vi "TimeSampleDlg.vi"() -> (1 "定时采样信息":string[][](array[string]), 2 "定时采样信息":T1, 3 "定时采样out":i32(listbox), 5 "是否采样":bool)   [LabVIEW 2014, in "Sample.lvlib"]
uses:
  Sample.lvlib
  DataBase/DataBase.lvlib
  DetectElecrodes/DetectElectros.lvlib
panel:
  out "编号":string
  in  "退出":bool
  in  "删除":bool
  in  "修改":bool
  in  "新增":bool
  in  "定时采样设置":i32(listbox)
  in  "退出":bool
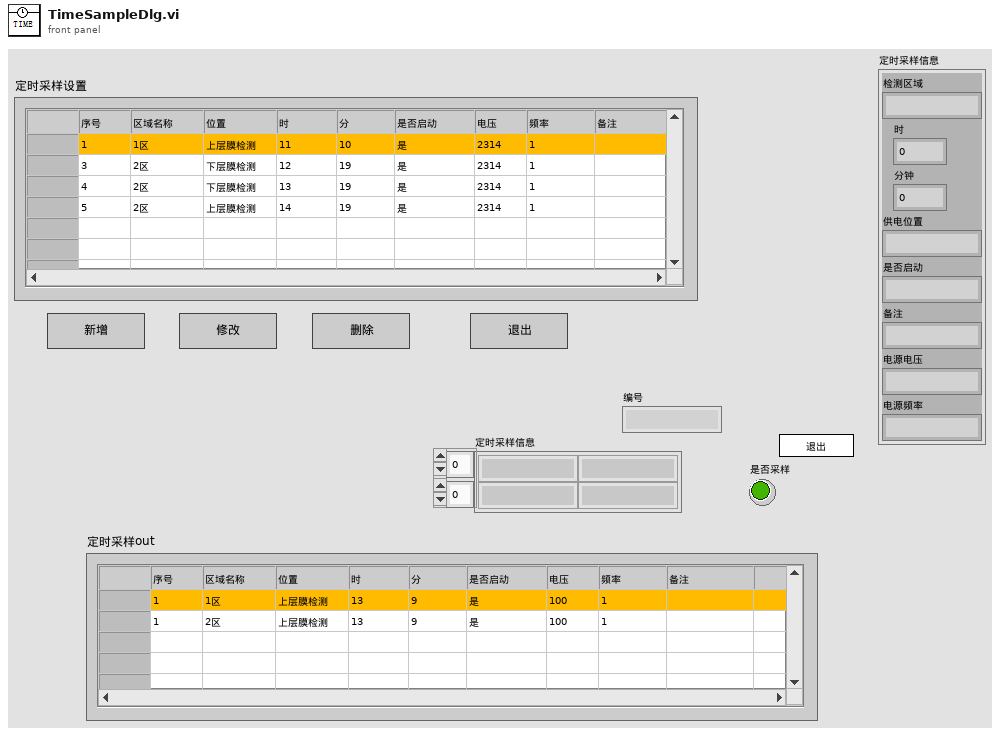
[diagram p1: front panel]
types:
  T1 = cluster{"检测区域":string, "时":u16, "分钟":u16, "供电位置":string, "是否启动":string, "备注":string, "电源电压":string, "电源频率":string}
  T2 = enum32{"invalid app kind", "Development System", "Run Time System", "Student Edition", "Embedded LabVIEW", "Evaluation", "Custom"}
  T3 = enum32{"Invalid", "Standard", "Closed", "Hidden", "Minimized", "Maximized"}
  T4 = cluster{"Core":cluster{"Current VI Reference":refnum<vi>, "Close Panel on Exit?":bool}, "Your Boolean data":bool, "Your string data":string, "定时采样信息":cluster{"检测区域":string, "时":u16, "分钟":u16, "供电位置":string, "是否启动":string, "备注":string, "电源电压":string, "电源频率":string}, "定时采样List":string[], "sampleSet记录":string[][], "Row":i32}
  T5 = typedef "LVPoint32TypeDef.ctl" = cluster{"Horizontal":i32, "Vertical":i32}
  T6 = typedef "LVRowAndColumnTypeDef.ctl" = cluster{"Row":i32, "Column":i32}
  T7 = cluster{"Current VI Reference":refnum<vi>, "Close Panel on Exit?":bool}
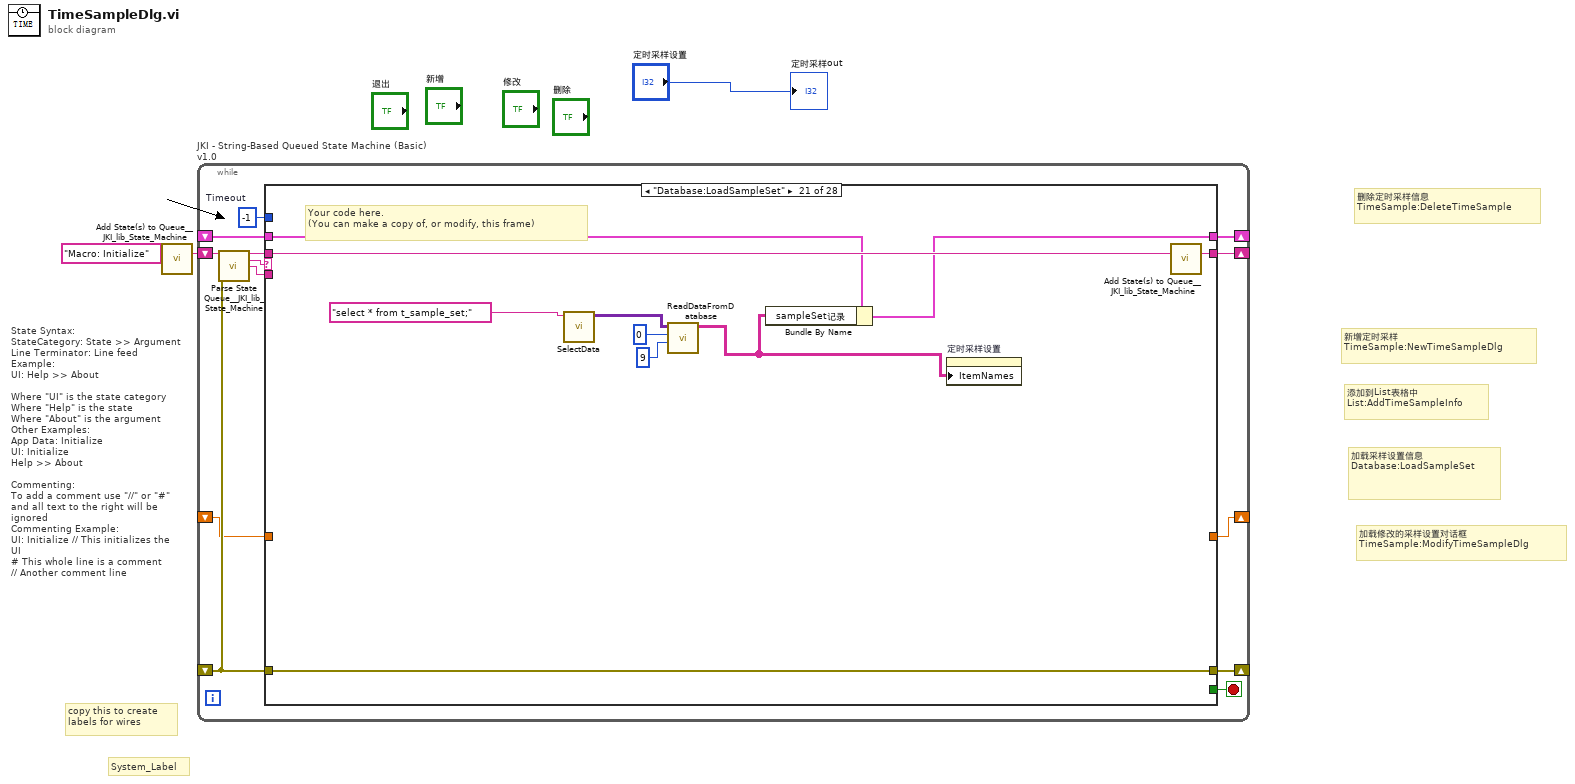
[diagram p0: block diagram]
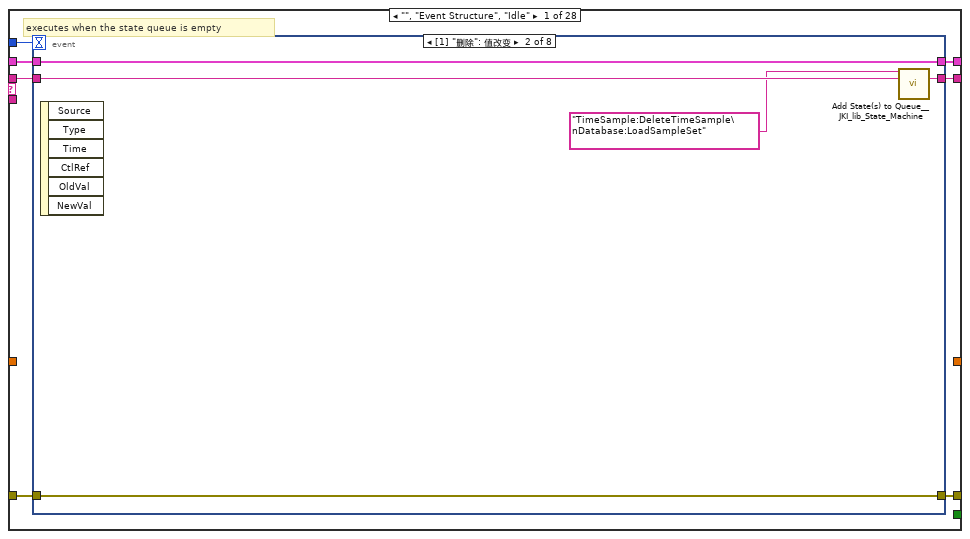
[diagram p2: hidden frame]
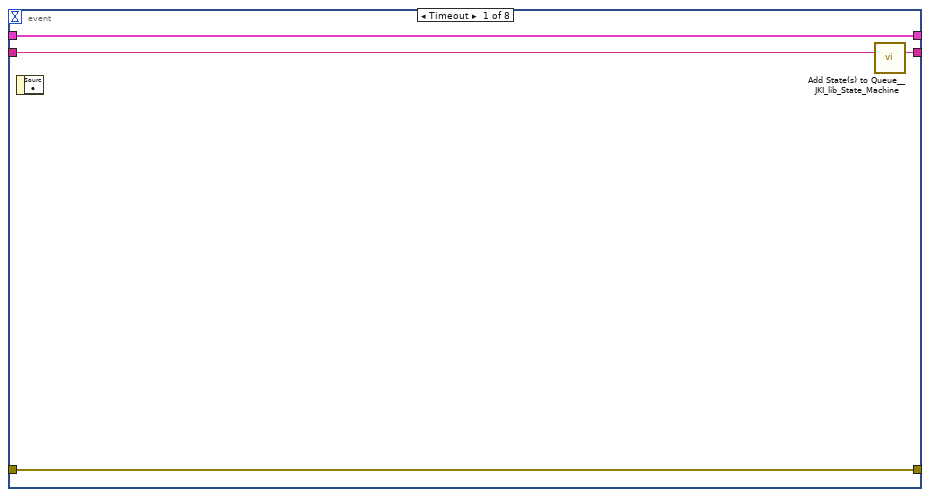
[diagram p3: hidden frame]
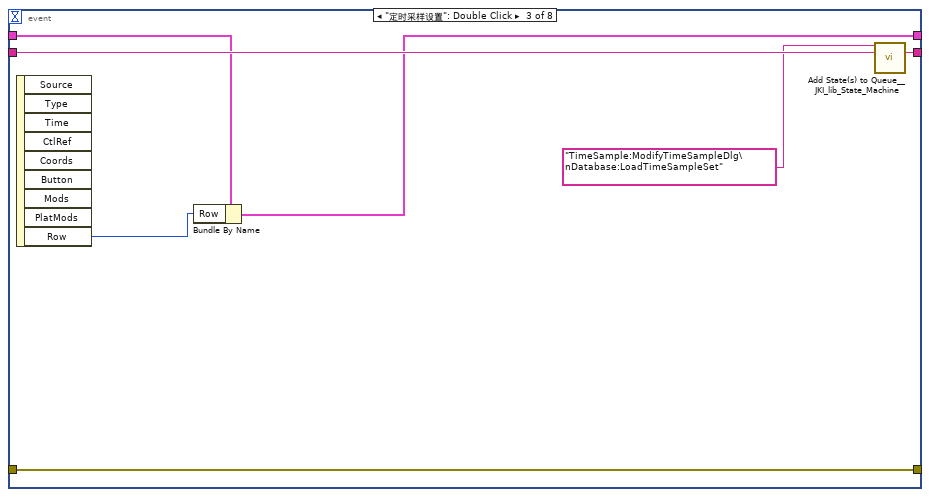
[diagram p4: hidden frame]
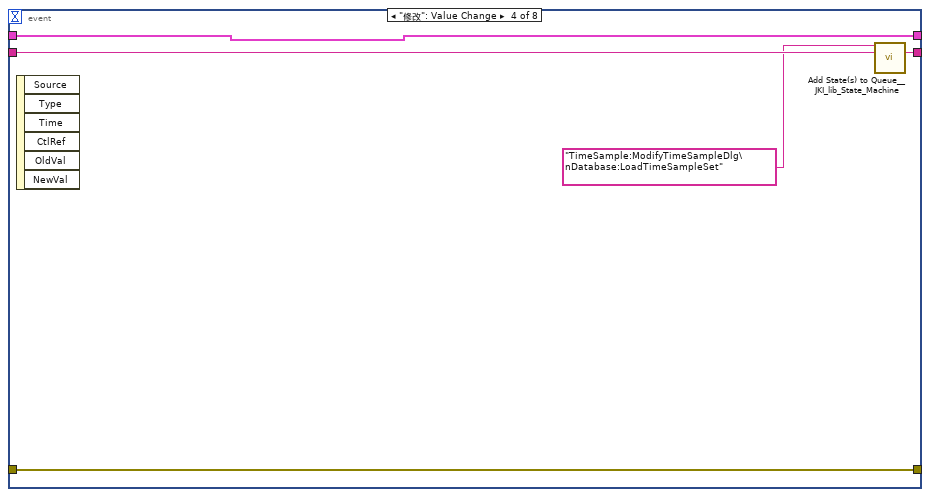
[diagram p5: hidden frame]
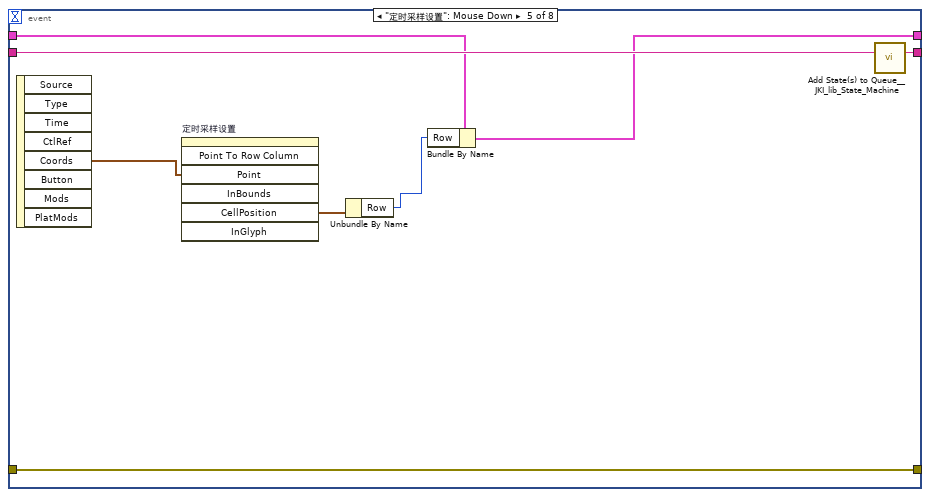
[diagram p6: hidden frame]
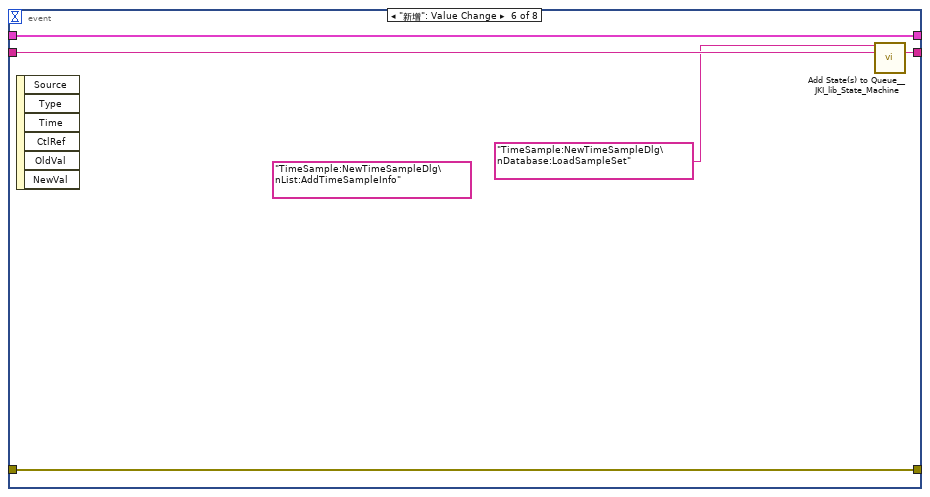
[diagram p7: hidden frame]
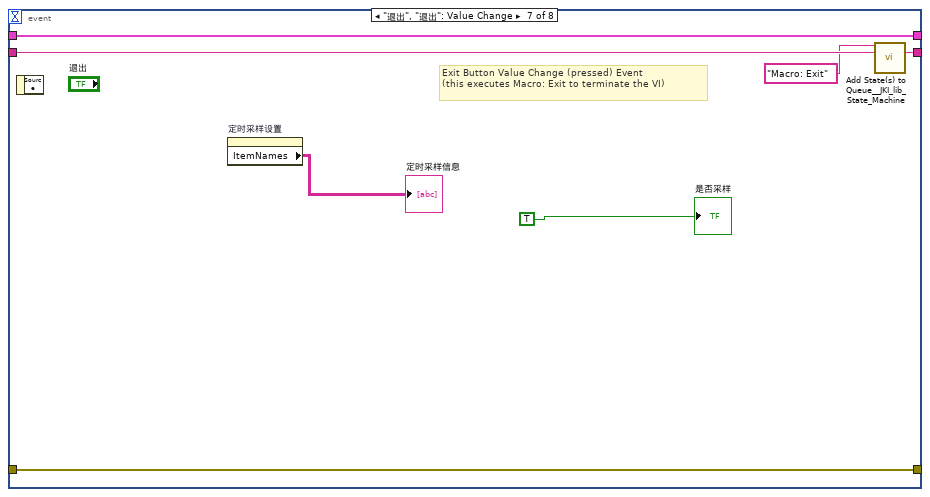
[diagram p8: hidden frame]
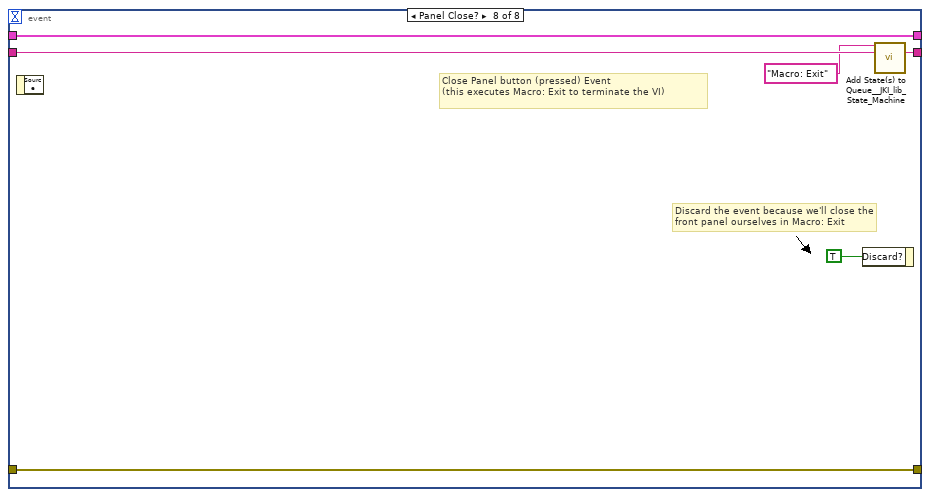
[diagram p9: hidden frame]
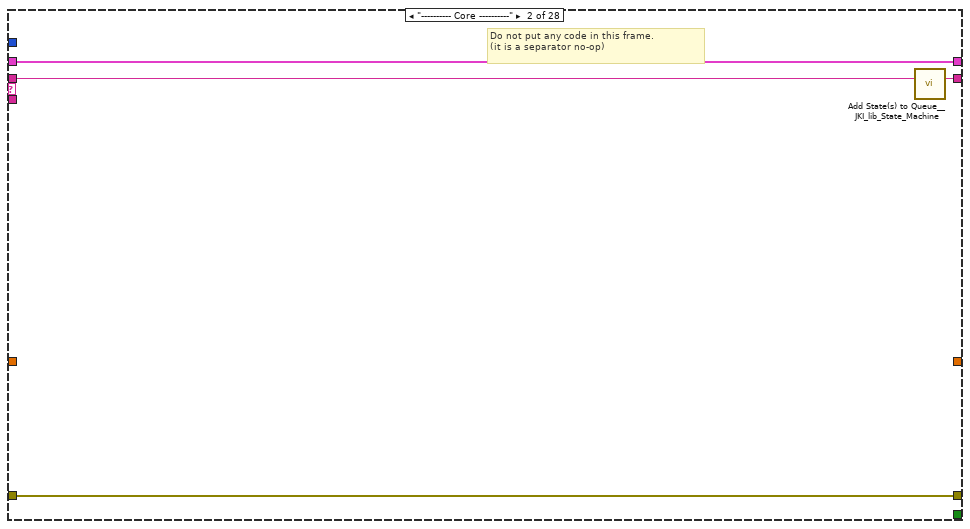
[diagram p10: hidden frame]
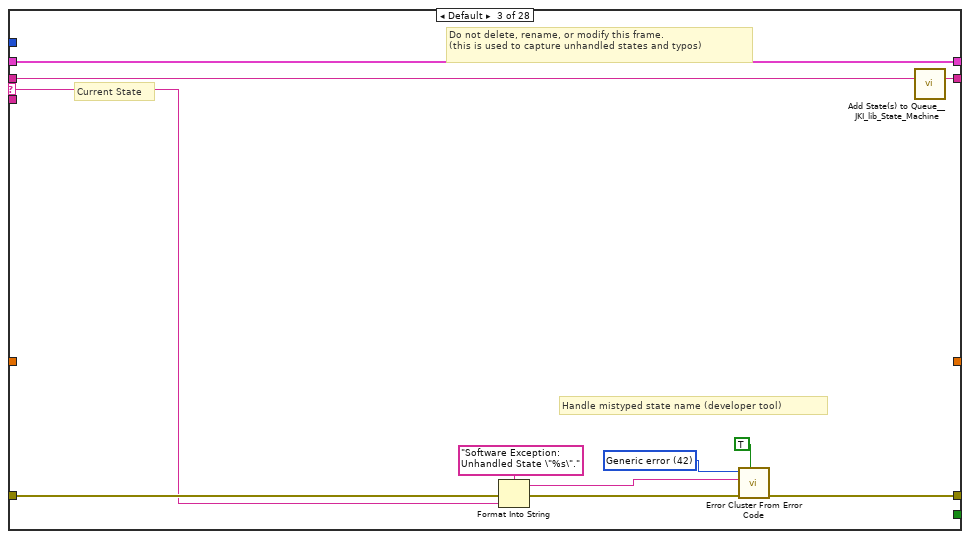
[diagram p11: hidden frame]
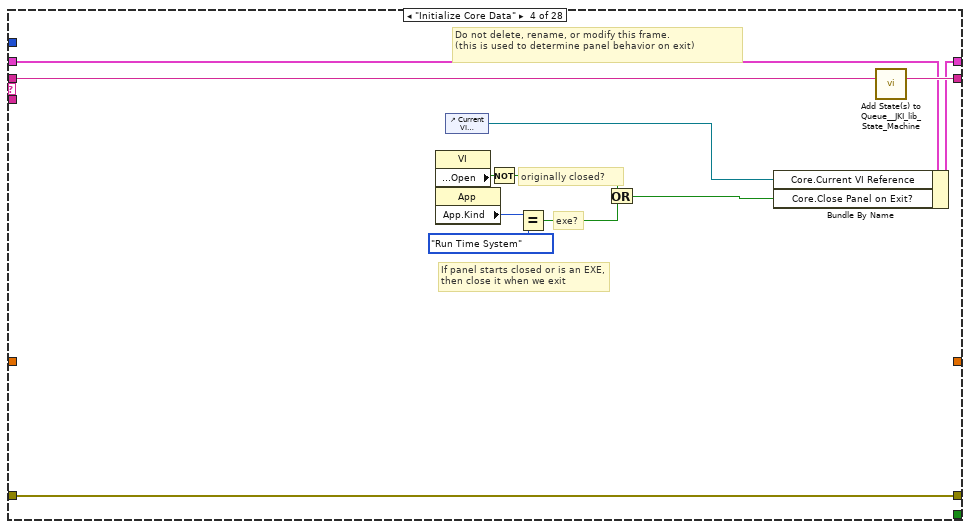
[diagram p12: hidden frame]
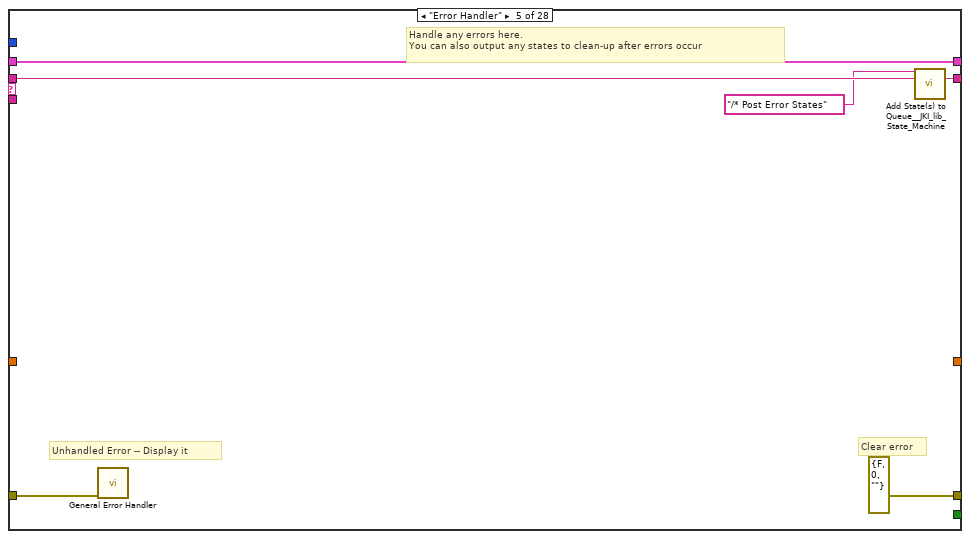
[diagram p13: hidden frame]
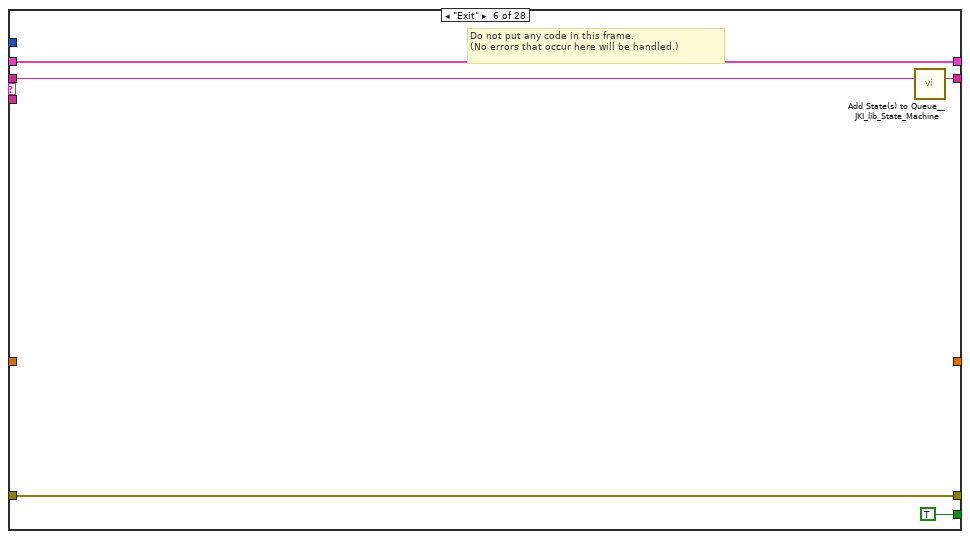
[diagram p14: hidden frame]
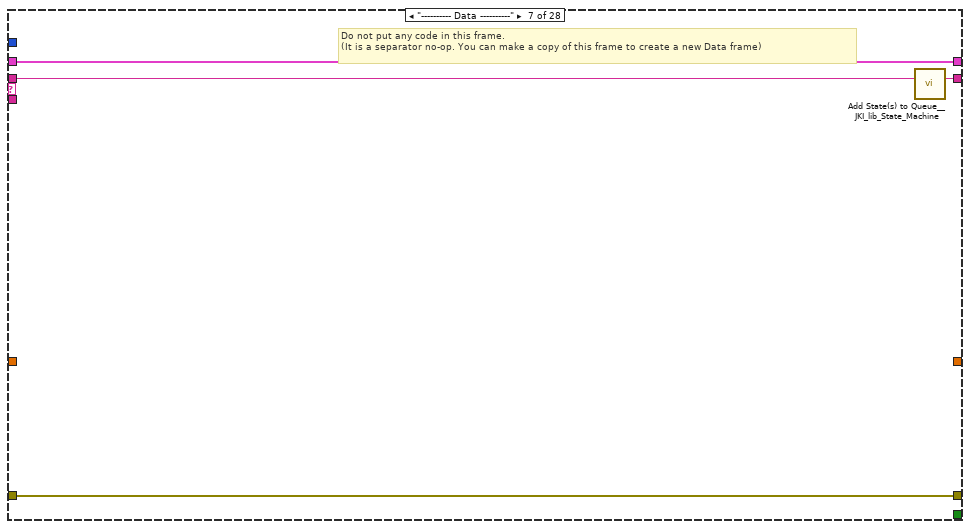
[diagram p15: hidden frame]
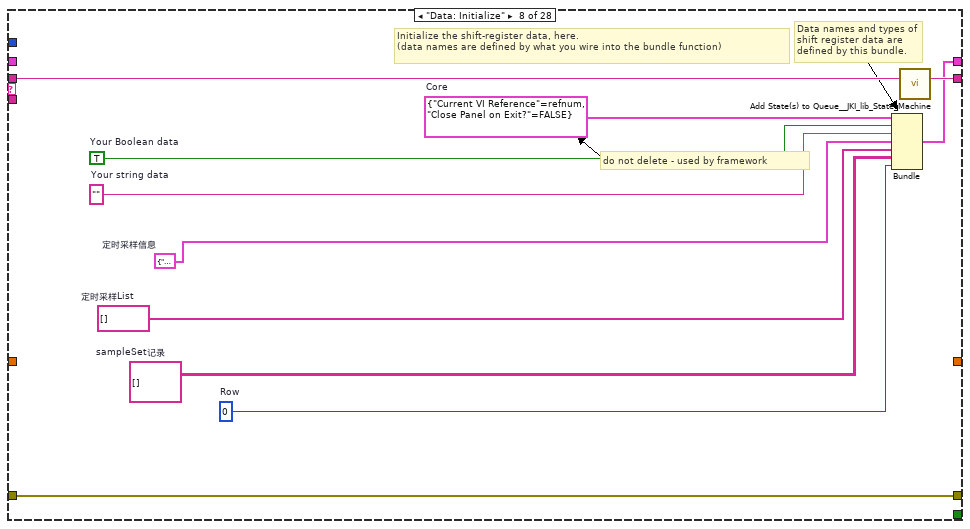
[diagram p16: hidden frame]
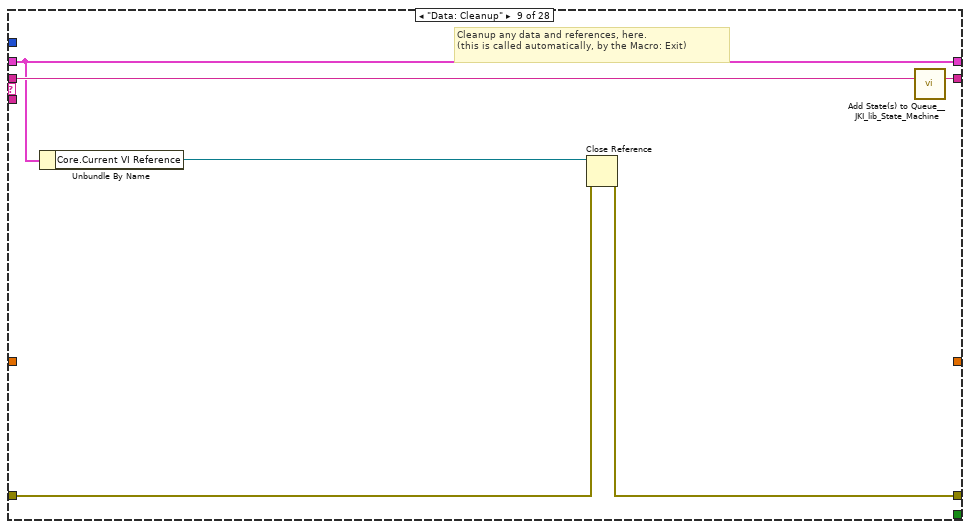
[diagram p17: hidden frame]
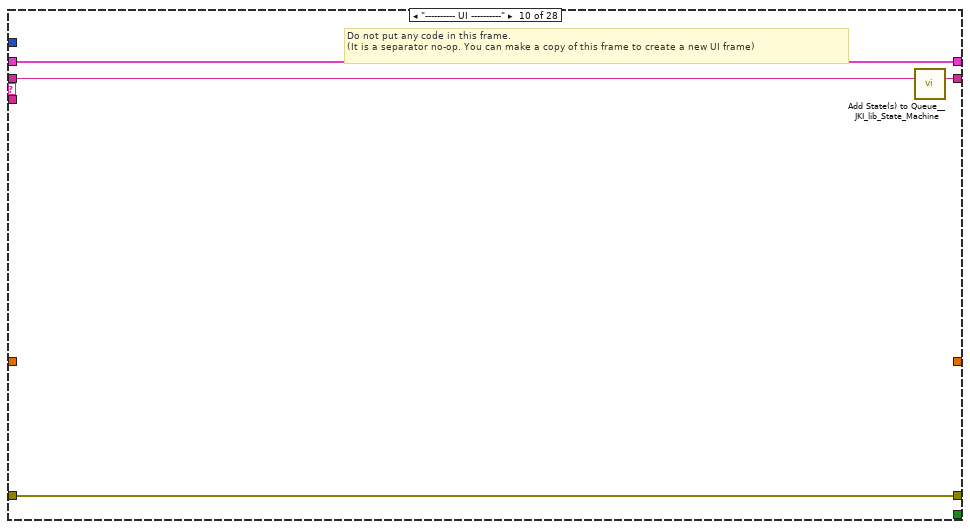
[diagram p18: hidden frame]
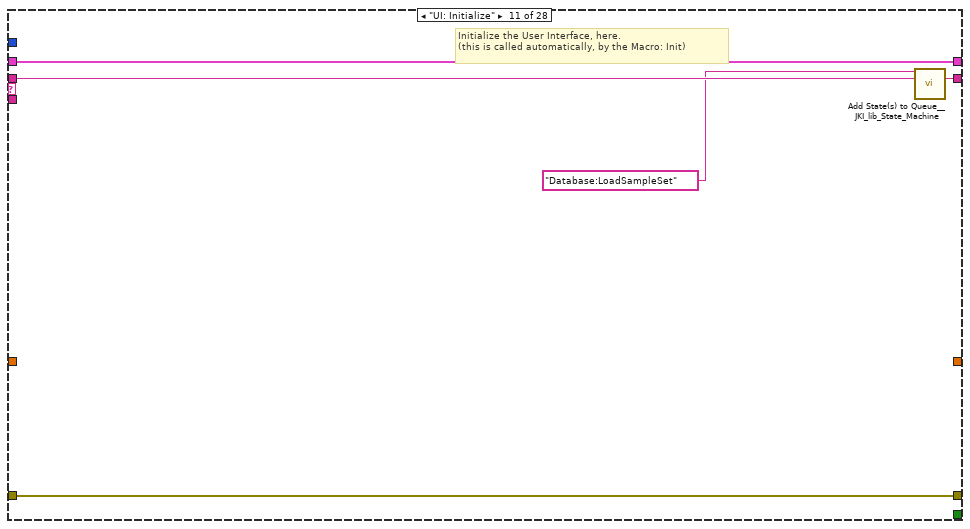
[diagram p19: hidden frame]
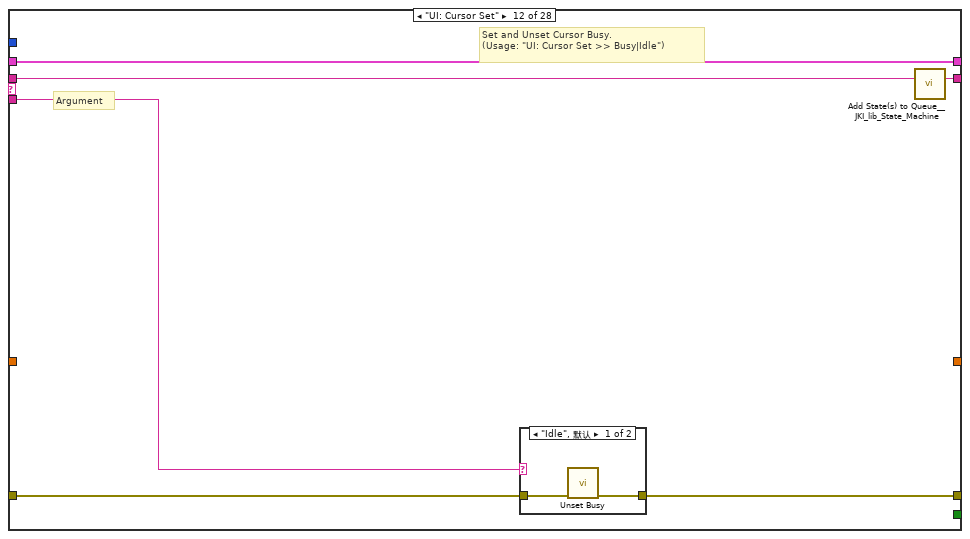
[diagram p20: hidden frame]
diagram:
  # "删除定时采样信息\nTimeSample:DeleteTimeSample"
  # "加载修改的采样设置对话框\nTimeSample:ModifyTimeSampleDlg"
  # "加载采样设置信息\nDatabase:LoadSampleSet"
  # "添加到List表格中\nList:AddTimeSampleInfo"
  # "新增定时采样\nTimeSample:NewTimeSampleDlg"
  # "State Syntax:\nStateCategory: State >> Argument\nLine Terminator: Line feed\nExample:\nUI: Help >> About\n\nWhere \"UI\" is the state category\nWhere \"Help\" is the state\nWhere \"About\" is the argument\nOther Examples:\nApp Data: Initialize\nUI: Initialize\nHelp >> About\n\nCommenting:\nTo add a comment use \"//\" or \"#\" and all text to the right will be ignored\nCommenting Example:\nUI: Initialize // This initializes the UI\n# This whole line is a comment\n// Another comment line"
  # "copy this to create labels for wires"
  # "System_Label"
  n1 = call <vilib>:"Add State(s) to Queue__JKI_lib_State_Machine.vi"("State(s) in (\"\")"="Macro: Initialize") -> ("States Out"=w3:string)  [unwired: 14 in]
  n2 = while "JKI - String-Based Queued State Machine (Basic) v1.0" {
    shift-right: [w9] -> _
    shift-left: _ -> [w8]
    shift-right: [w12] -> _
    shift-left: _ -> [w6]
    shift-right: [w11] -> _
    shift-left: w3 -> [w13]
    shift-right: [w4] -> _
    shift-left: _ -> [w5]
    stop <- w10 stop-if-true
    w7 = -1  # Timeout
    n3 = call <vilib>:"Parse State Queue__JKI_lib_State_Machine.vi"("State Queue"=w13, "Error In (no error)"=w6) -> ("Remaining States"=w15:string, "Current State"=w16:string, "Arguments"=w14:string)  [unwired: 11 in]
    n4 = case shown="\"Database:LoadSampleSet\"" w16 {
      selector: w16 -> [_ _ w75 _ _ _ _ _ _ _ _ _ _ _ _ _ _ _ _ _ _ _ _ _ _ _ _ _]
      tunnel: w15 -> [w23 w74 w79 w97 w103 w108 w112 w123 w129 w133 w138 w144 w155 w181 w186 w196 w200 w204 w208 w212 w222 w232 w236 w257 w261 w273 w302 w308]
      tunnel: w14 -> [_ _ _ _ _ _ _ _ _ _ _ w139 w149 _ _ _ _ _ _ _ _ _ _ _ _ _ _ _]
      tunnel: w8 -> [w21 w71 w77 w88 w100 w106 w109 _ w124 w130 w136 w142 w151 w178 w183 w193 w197 w201 w205 w209 w215 w225 w233 w240 w258 w270 w294 w305]
      tunnel: [w20 w72 w81 w94 errorcluster {"status"=FALSE, "code"=0, "source"=""} ("error out") w105 w110 w120 w125 w131 w135 w140 w152 w179 w184 w194 w198 w202 w206 w210 w220 w230 w234 w255 w259 w271 w300 w306] -> w12
      tunnel: w6 -> [w19 w72 w80 w94 w99 w105 w110 w120 w126 w131 w135 w141 w153 w179 w184 w194 w198 w202 w206 w210 w220 w230 w234 w255 w259 w271 w300 w306]
      tunnel: [w22 w73 w78 w96 w102 w107 w111 w122 w128 w132 w137 w143 w154 w180 w185 w195 w199 w203 w207 w211 w221 w231 w235 w256 w260 w272 w301 w307] -> w11
      tunnel: [_ _ _ _ _ TRUE _ _ _ _ _ _ _ _ _ _ _ _ _ _ _ _ _ _ _ _ _ _] -> w10
      tunnel: [w18 w71 w77 w95 w100 w106 w109 w121 w124 w130 w136 w142 w151 w178 w183 w193 w197 w201 w205 w209 w214 w224 w233 w239 w258 w270 w294 w304] -> w9
      tunnel: w7 -> [w17 _ _ _ _ _ _ _ _ _ _ _ _ _ _ _ _ _ _ _ _ _ _ _ _ _ _ _]
      tunnel: w5 -> [_ _ _ _ _ _ _ _ _ _ _ _ _ _ _ _ _ _ _ _ _ _ _ w253 _ w262 _ _]
      tunnel: [_ _ _ _ _ _ _ _ _ _ _ _ _ _ _ _ _ _ _ _ _ _ _ w252 _ w262 _ _] -> w4
      frame "", "Event Structure", "Idle" {
        # "executes when the state queue is empty"
        n5 = event shown="[1] \"删除\": 值改变" {
          selector: _ -> [_ _ _ _ _ _ _ _]
          dyn-events: _ -> [_ _ _ _ _ _ _ _]
          timeout: w17 -> [_ _ _ _ _ _ _ _]
          tunnel: w23 -> [w27 w32 w39 w44 w52 w57 w64 w70]
          tunnel: [w26 w31 w38 w43 w51 w56 w63 w69] -> w22
          tunnel: w21 -> [w24 w29 w35 w40 w46 w54 w61 w67]
          tunnel: [w25 w30 w37 w42 w50 w55 w62 w68] -> w20
          tunnel: w19 -> [w25 w30 w37 w42 w50 w55 w62 w68]
          tunnel: [w24 w29 w34 w40 w45 w54 w61 w67] -> w18
          event Timeout {
            n6 = event-data() -> ()  [unwired: 1 in, 1 out]
            n7 = call <vilib>:"Add State(s) to Queue__JKI_lib_State_Machine.vi"("State(s) in (\"\")"=w27) -> ("States Out"=w26:string)  [unwired: 14 in]
          }
          event "删除": Value Change {
            n8 = event-data() -> ()  [unwired: 1 in, 6 out]
            n9 = call <vilib>:"Add State(s) to Queue__JKI_lib_State_Machine.vi"("State(s) in Front (\"\")"="TimeSample:DeleteTimeSample\nDatabase:LoadSampleSet", "State(s) in (\"\")"=w32) -> ("States Out"=w31:string)  [unwired: 13 in]
          }
          event "定时采样设置": Double Click {
            n10 = event-data() -> ("Row"=w36:i32)  [unwired: 1 in, 8 out]
            n11 = Bundle By Name(cluster=w35, "Row"=w36) -> (w34:T4)
            n12 = call <vilib>:"Add State(s) to Queue__JKI_lib_State_Machine.vi"("State(s) in Front (\"\")"="TimeSample:ModifyTimeSampleDlg\nDatabase:LoadTimeSampleSet", "State(s) in (\"\")"=w39) -> ("States Out"=w38:string)  [unwired: 13 in]
          }
          event "修改": Value Change {
            n13 = event-data() -> ()  [unwired: 1 in, 6 out]
            n14 = call <vilib>:"Add State(s) to Queue__JKI_lib_State_Machine.vi"("State(s) in Front (\"\")"="TimeSample:ModifyTimeSampleDlg\nDatabase:LoadTimeSampleSet", "State(s) in (\"\")"=w44) -> ("States Out"=w43:string)  [unwired: 13 in]
          }
          event "定时采样设置": Mouse Down {
            n15 = event-data() -> ("Coords"=w49:T5)  [unwired: 1 in, 7 out]
            n16 = invoke on="定时采样设置" class="MCListbox (严格)" method="Point To Row Column"("Point"=w49) -> ("CellPosition"=w48:T6)  [unwired: 6 in, 6 out]
            n17 = Unbundle By Name(w48) -> ("Row"=w47:i32)
            n18 = Bundle By Name(cluster=w46, "Row"=w47) -> (w45:T4)
            n19 = call <vilib>:"Add State(s) to Queue__JKI_lib_State_Machine.vi"("State(s) in (\"\")"=w52) -> ("States Out"=w51:string)  [unwired: 14 in]
          }
          event "新增": Value Change {
            (unwired) "TimeSample:NewTimeSampleDlg\nList:AddTimeSampleInfo"
            n20 = event-data() -> ()  [unwired: 1 in, 6 out]
            n21 = call <vilib>:"Add State(s) to Queue__JKI_lib_State_Machine.vi"("State(s) in Front (\"\")"="TimeSample:NewTimeSampleDlg\nDatabase:LoadSampleSet", "State(s) in (\"\")"=w57) -> ("States Out"=w56:string)  [unwired: 13 in]
          }
          event "退出", "退出": Value Change {
            # "Exit Button Value Change (pressed) Event\n(this executes Macro: Exit to terminate the VI)"
            n22 = event-data() -> ()  [unwired: 1 in, 1 out]
            n23 = property on="定时采样设置" class="MCListbox (严格)"() -> ("ItemNames"=→"定时采样信息":string[][])  [unwired: 2 in, 2 out]
            n24 = call <vilib>:"Add State(s) to Queue__JKI_lib_State_Machine.vi"("State(s) in Front (\"\")"="Macro: Exit", "State(s) in (\"\")"=w64) -> ("States Out"=w63:string)  [unwired: 13 in]
            "是否采样" <- TRUE
          }
          event Panel Close? {
            # "Discard the event because we'll close the front panel ourselves in Macro: Exit"
            # "Close Panel button (pressed) Event\n(this executes Macro: Exit to terminate the VI)"
            n25 = event-data() -> ()  [unwired: 1 in, 1 out]
            n26 = event-data("Discard?"=TRUE) -> ()  [unwired: 1 in, 1 out]
            n27 = call <vilib>:"Add State(s) to Queue__JKI_lib_State_Machine.vi"("State(s) in Front (\"\")"="Macro: Exit", "State(s) in (\"\")"=w70) -> ("States Out"=w69:string)  [unwired: 13 in]
          }
        }
      }
      frame "---------- Core ----------" {
        # "Do not put any code in this frame.\n(it is a separator no-op)"
        n28 = call <vilib>:"Add State(s) to Queue__JKI_lib_State_Machine.vi"("State(s) in (\"\")"=w74) -> ("States Out"=w73:string)  [unwired: 14 in]
      }
      frame Default {
        w84 = 42 items=["No error", "Argument error", "Memory is full", "Out of zone", "End of file", "File already open", "Generic file I/O error", "File not found", "File permission error", "Disk is full", "Duplicate path", "Too many files open", "System feature not enabled", "Resource file not found", "Cannot add resource", "Resource not found", "Image not found", "Image memory error", "Pen does not exist", "Config type invalid", "Config token not found", "Config parse error", "Config memory error", "Bad external code format", "Bad external code offset", "External code not present", "Null window", "Destroy window error", "Null menu", "Print aborted", "Bad print record", "Print driver error", "Windows error during printing", "Memory error during printing", "Print dialog error", "Generic print error", "Invalid device refnum", "Device not found", "Device parameter error", "Device unit error", "Cannot open device", "Device call aborted", "Generic error", "Cancelled by user", "Object ID too low", "Object ID too high", "Object not in heap", "Unknown heap", "Unknown object (invalid DefProc)", "Unknown object (DefProc not in table)", "Message out of range", "Invalid (null) method", "Unknown message", "Manager call not supported", "Bad address", "Network operation in progress", "Network operation timed out", "Connection is busy", "Network attribute not supported", "Network error", "Address in use", "System out of memory", "Connection aborted", "Connection refused", "Not connected", "Already connected", "Connection closed", "Initialization error (interapplication manager)", "Bad occurrence", "Wait on unbound occurrence handler", "Occurrence queue overflow", "Datalog type conflict", "Unused", "Unrecognized type (interapplication manager)", "Memory corrupt", "Failed to make temporary DLL", "Old CIN version", "Drag socket not found", "Failed to load drop-object", "Failed to register OLE object", "Failed to release OLE object", "Format specifier type mismatch", "Unknown format specifier", "Too few format specifiers", "Too many format specifiers", "Scan failed", "Newer CIN version", "Error converting to variant", "Runtime menu error", "Password tampered", "Variant attribute not found", "Incompatible variant data type", "Event data is not available", "Event Store is not present", "Occurrence is not found", "Event Queue is not created", "Event info is not available", "Refnum passed is NULL", "Error retrieving Class GUID", "Error retrieving CoClass GUID", "Error retrieving TypeLib GUID.", "Bad built application magic bytes.", "Specific driver is different from the specific driver associated with the Logical Name.", "There is no session opened to the class driver.", "Max Error", "MAX - Error with config objects", "MAX - Error loading configuration", "MAX - Group not supported"]
        # "Current State"
        # "Do not delete, rename, or modify this frame.\n(this is used to capture unhandled states and typos)"
        # "Handle mistyped state name (developer tool)"
        n29 = Format Into String(format string="Software Exception: Unhandled State \"%s\"." ("message"), error in=w80, w75) -> (resulting string=w83:string, error out=w82:errorcluster)  [unwired: 1 in]
        n30 = call <vilib>:"Error Cluster From Error Code.vi"("show call chain? (False)"=TRUE, "error in (no error)"=w82, "error message (\"\")"=w83, "error code (0)"=w84) -> ("error out"=w81:errorcluster)  [unwired: 5 in]
        n31 = call <vilib>:"Add State(s) to Queue__JKI_lib_State_Machine.vi"("State(s) in (\"\")"=w79) -> ("States Out"=w78:string)  [unwired: 14 in]
      }
      frame "Initialize Core Data" {
        # "Do not delete, rename, or modify this frame.\n(this is used to determine panel behavior on exit)"
        # "originally closed?"
        # "exe?"
        # "If panel starts closed or is an EXE, then close it when we exit"
        n32 = property class="VI"() -> ("Front Panel.Open"=w93:bool)  [unwired: 2 in, 2 out]
        n33 = property class="App"() -> ("App.Kind"=w92:T2)  [unwired: 2 in, 2 out]
        n34 = control-ref of="Current VI Reference"() -> (w86:refnum<vi>)
        n35 = Not(x=w93) -> (.not. x?=w90:bool)
        n36 = Equal?(x=w92, y=T2."Run Time System" ("Application:Kind")) -> (x = y?=w89:bool)
        n37 = Or(x=w90, y=w89) -> (x .or. y?=w87:bool)
        n38 = Bundle By Name(cluster=w88, "Core.Current VI Reference"=w86, "Core.Close Panel on Exit?"=w87) -> (w95:T4)
        n39 = call <vilib>:"Add State(s) to Queue__JKI_lib_State_Machine.vi"("State(s) in (\"\")"=w97) -> ("States Out"=w96:string)  [unwired: 14 in]
      }
      frame "Error Handler" {
        # "Unhandled Error -- Display it"
        # "Handle any errors here.\nYou can also output any states to clean-up after errors occur"
        # "Clear error"
        n40 = call <vilib>:"General Error Handler.vi"("error in (no error)"=w99) -> ()  [unwired: 10 in, 5 out]
        n41 = call <vilib>:"Add State(s) to Queue__JKI_lib_State_Machine.vi"("State(s) in Front (\"\")"="/* Post Error States", "State(s) in (\"\")"=w103) -> ("States Out"=w102:string)  [unwired: 13 in]
      }
      frame "Exit" {
        # "Do not put any code in this frame.\n(No errors that occur here will be handled.)"
        n42 = call <vilib>:"Add State(s) to Queue__JKI_lib_State_Machine.vi"("State(s) in (\"\")"=w108) -> ("States Out"=w107:string)  [unwired: 14 in]
      }
      frame "---------- Data ----------" {
        # "Do not put any code in this frame.\n(It is a separator no-op. You can make a copy of this frame to create a new Data frame)"
        n43 = call <vilib>:"Add State(s) to Queue__JKI_lib_State_Machine.vi"("State(s) in (\"\")"=w112) -> ("States Out"=w111:string)  [unwired: 14 in]
      }
      frame "Data: Initialize" {
        w113 = 0  # Row
        w114 = string[][] []  # sampleSet记录
        w115 = string[] []  # 定时采样List
        w116 = T1 {"检测区域"="", "时"=0, "分钟"=0, "供电位置"="", "是否启动"="", "备注"="", "电源电压"="", "电源频率"=""}  # 定时采样信息
        w117 = T7 {"Current VI Reference"=refnum, "Close Panel on Exit?"=FALSE}  # Core
        w119 = TRUE  # Your Boolean data
        w118 = ""  # Your string data
        # "do not delete - used by framework"
        # "Data names and types of shift register data are defined by this bundle."
        # "Initialize the shift-register data, here.\n(data names are defined by what you wire into the bundle function)"
        n44 = Bundle("Core"=w117, "Your Boolean data"=w119, "Your string data"=w118, "定时采样信息"=w116, "定时采样List"=w115, "sampleSet记录"=w114, "Row"=w113) -> (w121:T4)  [unwired: 1 in]
        n45 = call <vilib>:"Add State(s) to Queue__JKI_lib_State_Machine.vi"("State(s) in (\"\")"=w123) -> ("States Out"=w122:string)  [unwired: 14 in]
      }
      frame "Data: Cleanup" {
        # "Cleanup any data and references, here.\n(this is called automatically, by the Macro: Exit)"
        n46 = Unbundle By Name(w124) -> ("Core.Current VI Reference"=w127:refnum<vi>)
        n47 = Close Reference(reference=w127, error in (no error)=w126) -> (error out=w125:errorcluster)
        n48 = call <vilib>:"Add State(s) to Queue__JKI_lib_State_Machine.vi"("State(s) in (\"\")"=w129) -> ("States Out"=w128:string)  [unwired: 14 in]
      }
      frame "---------- UI ----------" {
        # "Do not put any code in this frame.\n(It is a separator no-op. You can make a copy of this frame to create a new UI frame)"
        n49 = call <vilib>:"Add State(s) to Queue__JKI_lib_State_Machine.vi"("State(s) in (\"\")"=w133) -> ("States Out"=w132:string)  [unwired: 14 in]
      }
      frame "UI: Initialize" {
        # "Initialize the User Interface, here.\n(this is called automatically, by the Macro: Init)"
        n50 = call <vilib>:"Add State(s) to Queue__JKI_lib_State_Machine.vi"("State(s) in Front (\"\")"="Database:LoadSampleSet", "State(s) in (\"\")"=w138) -> ("States Out"=w137:string)  [unwired: 13 in]
      }
      frame "UI: Cursor Set" {
        # "Argument"
        # "Set and Unset Cursor Busy.\n(Usage: \"UI: Cursor Set >> Busy|Idle\")"
        n51 = case shown="\"Idle\", 默认" w139 {
          tunnel: w141 -> [w146 w148]
          tunnel: [w145 w147] -> w140
          frame "Idle", Default {
            n52 = call <vilib>:"Unset Busy.vi"("error in (no error)"=w146) -> ("error out"=w145:errorcluster)  [unwired: 10 in]
          }
          frame "Busy" {
            n53 = call <vilib>:"Set Busy.vi"("error in (no error)"=w148) -> ("error out"=w147:errorcluster)  [unwired: 9 in, 1 out]
          }
        }
        n54 = call <vilib>:"Add State(s) to Queue__JKI_lib_State_Machine.vi"("State(s) in (\"\")"=w144) -> ("States Out"=w143:string)  [unwired: 14 in]
      }
      frame "UI: Front Panel State" {
        # "Argument"
        # "Set Front Panel Open or Closed\n(Usage: \"UI: Front Panel State >> Open|Close\")"
        n55 = Unbundle By Name(w151) -> ("Core.Current VI Reference"=w150:refnum<vi>)
        n56 = case shown="\"Open\", 默认" w149 {
          tunnel: w153 -> [w159 w172]
          tunnel: [w161 w173] -> w152
          tunnel: w150 -> [w160 w170]
          frame "Open", Default {
            n57 = property class="VI"(reference=w160, error in=w159) -> (reference out=w157:refnum<vi>, error out=w158:errorcluster, "Front Panel.Open"=w156:bool)
            n58 = case shown="假" w156 {
              tunnel: [w164 w167] -> w161
              tunnel: w158 -> [w163 w167]
              tunnel: w157 -> [w162 _]
              frame False {
                n59 = invoke class="VI" method="FP.Open"(reference=w162, error in=w163, "Activate"=TRUE, "State"=T3."Standard") -> (error out=w164:errorcluster)  [unwired: 1 in, 4 out]
              }
              frame True {
              }
            }
          }
          frame "Close" {
            n60 = property class="VI"(reference=w170, error in=w172) -> (reference out=w169:refnum<vi>, error out=w171:errorcluster, "Front Panel.Open"=w168:bool)
            n61 = case shown="真" w168 {
              tunnel: [w174 w177] -> w173
              tunnel: w171 -> [w174 w176]
              tunnel: w169 -> [_ w175]
              frame False {
              }
              frame True {
                n62 = invoke class="VI" method="FP.Close"(reference=w175, error in=w176) -> (error out=w177:errorcluster)  [unwired: 1 in, 2 out]
              }
            }
          }
        }
        n63 = call <vilib>:"Add State(s) to Queue__JKI_lib_State_Machine.vi"("State(s) in (\"\")"=w155) -> ("States Out"=w154:string)  [unwired: 14 in]
      }
      frame "---------- Macro ----------" {
        # "Do not put any code in this frame.\n(It is a separator no-op. You can make a copy of this frame to create a new Macro frame)"
        n64 = call <vilib>:"Add State(s) to Queue__JKI_lib_State_Machine.vi"("State(s) in (\"\")"=w181) -> ("States Out"=w180:string)  [unwired: 14 in]
      }
      frame "Macro: Initialize" {
        w182 = "Data: Initialize\nInitialize Core Data\nUI: Initialize\nUI: Front Panel State >> Open"  # Data: Initialize Initialize Core Data UI: Initialize UI: Front Panel State >> Open
        # "Initialization Macro\n(This is called once, when the VI starts)"
        n65 = call <vilib>:"Add State(s) to Queue__JKI_lib_State_Machine.vi"("State(s) in Front (\"\")"=w182, "State(s) in (\"\")"=w186) -> ("States Out"=w185:string)  [unwired: 13 in]
      }
      frame "Macro: Exit" {
        # "Exit Macro\n(This is called once, when the VI exits)"
        n66 = Unbundle By Name(w193) -> ("Core.Close Panel on Exit?"=w192:bool)
        n67 = Select(t="UI: Front Panel State >> Close", s=w192, f="") -> (s? t:f=w189:string)
        n68 = call <vilib>:"Add State(s) to Queue__JKI_lib_State_Machine.vi"("State(s) in (\"\")"=w189, "State(s) at Back (\"\")"="Data: Cleanup\nExit") -> ("States Out"=w187:string)  [unwired: 13 in]
        n69 = call <vilib>:"Add State(s) to Queue__JKI_lib_State_Machine.vi"("State(s) in Front (\"\")"=w187, "State(s) in (\"\")"=w196) -> ("States Out"=w195:string)  [unwired: 13 in]
      }
      frame "---------- New Category ----------" {
        # "Template Separator\n(You can make a copy of, or modify, this frame)"
        n70 = call <vilib>:"Add State(s) to Queue__JKI_lib_State_Machine.vi"("State(s) in (\"\")"=w200) -> ("States Out"=w199:string)  [unwired: 14 in]
      }
      frame "New Category: 1" {
        # "Your code here.\n(You can make a copy of, or modify, this frame)"
        n71 = call <vilib>:"Add State(s) to Queue__JKI_lib_State_Machine.vi"("State(s) in (\"\")"=w204) -> ("States Out"=w203:string)  [unwired: 14 in]
      }
      frame "New Category: 2" {
        # "Your code here.\n(You can make a copy of, or modify, this frame)"
        n72 = call <vilib>:"Add State(s) to Queue__JKI_lib_State_Machine.vi"("State(s) in (\"\")"=w208) -> ("States Out"=w207:string)  [unwired: 14 in]
      }
      frame "----------Database--------" {
        # "Your code here.\n(You can make a copy of, or modify, this frame)"
        n73 = call <vilib>:"Add State(s) to Queue__JKI_lib_State_Machine.vi"("State(s) in (\"\")"=w212) -> ("States Out"=w211:string)  [unwired: 14 in]
      }
      frame "Database:LoadSampleSet" {
        # "Your code here.\n(You can make a copy of, or modify, this frame)"
        n74 = call "SelectData.vi"("SQL query"="select * from t_sample_set;") -> ("recordset data"=w218:variant[][])  [unwired: 7 in, 1 out]
        n75 = call "ReadDataFromDatabase.vi"("长度"=9, "index"=0, "recordset data"=w218) -> ("所有记录"=w213:string[][])  [unwired: 7 in, 1 out]
        n76 = Bundle By Name(cluster=w215, "sampleSet记录"=w213) -> (w214:T4)
        n77 = property on="定时采样设置" class="MCListbox (严格)"("ItemNames"=w213) -> ()  [unwired: 2 in, 2 out]
        n78 = call <vilib>:"Add State(s) to Queue__JKI_lib_State_Machine.vi"("State(s) in (\"\")"=w222) -> ("States Out"=w221:string)  [unwired: 14 in]
      }
      frame "Database:LoadTimeSampleSet" {
        # "Your code here.\n(You can make a copy of, or modify, this frame)"
        n79 = call "SelectData.vi"("SQL query"="select * from t_sample_set;") -> ("recordset data"=w228:variant[][])  [unwired: 7 in, 1 out]
        n80 = call "ReadDataFromDatabase.vi"("长度"=9, "index"=0, "recordset data"=w228) -> ("所有记录"=w223:string[][])  [unwired: 7 in, 1 out]
        n81 = Bundle By Name(cluster=w225, "sampleSet记录"=w223) -> (w224:T4)
        n82 = property on="定时采样设置" class="MCListbox (严格)"("ItemNames"=w223) -> ()  [unwired: 2 in, 2 out]
        n83 = call <vilib>:"Add State(s) to Queue__JKI_lib_State_Machine.vi"("State(s) in (\"\")"=w232) -> ("States Out"=w231:string)  [unwired: 14 in]
      }
      frame "------------List--------" {
        # "Your code here.\n(You can make a copy of, or modify, this frame)"
        n84 = call <vilib>:"Add State(s) to Queue__JKI_lib_State_Machine.vi"("State(s) in (\"\")"=w236) -> ("States Out"=w235:string)  [unwired: 14 in]
      }
      frame "List:AddTimeSampleInfo" {
        # "没有使用的状态"
        n85 = Unbundle By Name(w240) -> ("定时采样信息.检测区域"=w250:string, "定时采样信息.时"=w248:u16, "定时采样信息.分钟"=w247:u16, "定时采样信息.供电位置"=w249:string, "定时采样信息.是否启动"=w244:string, "定时采样信息.备注"=w241:string, "定时采样信息.电源电压"=w243:string, "定时采样信息.电源频率"=w242:string, "定时采样信息"=→"定时采样信息":T1)
        n86 = Increment(x=w253) -> (x+1=w252:dbl)
        n87 = Number To Decimal String(number=w252) -> (decimal integer string=w251:string)  [unwired: 1 in]
        n88 = Number To Decimal String(number=w247) -> (decimal integer string=w245:string)  [unwired: 1 in]
        n89 = Number To Decimal String(number=w248) -> (decimal integer string=w246:string)  [unwired: 1 in]
        n90 = Build Array(w251, w250, w249, w246, w245, w244, w243, w242, w241) -> (w238:string[])
        n91 = Unbundle By Name(w240) -> ("定时采样List"=w237:string[])
        n92 = Bundle By Name(cluster=w240, "定时采样List"=w238) -> (w239:T4)
        n93 = Build Array(w237, w238) -> ()  [unwired: 1 out]
        n94 = call <vilib>:"Add State(s) to Queue__JKI_lib_State_Machine.vi"("State(s) in (\"\")"=w257) -> ("States Out"=w256:string)  [unwired: 14 in]
      }
      frame "----------TimeSample--------" {
        # "Your code here.\n(You can make a copy of, or modify, this frame)"
        n95 = call <vilib>:"Add State(s) to Queue__JKI_lib_State_Machine.vi"("State(s) in (\"\")"=w261) -> ("States Out"=w260:string)  [unwired: 14 in]
      }
      frame "TimeSample:DeleteTimeSample" {
        # "Your code here.\n(You can make a copy of, or modify, this frame)"
        n96 = Unbundle By Name(w270) -> ("Row"=w268:i32)
        n97 = property on="定时采样设置" class="MCListbox (严格)"() -> ("ItemNames"=w269:string[][])  [unwired: 2 in, 2 out]
        n98 = Index Array(array=w269, index (row)=w268) -> (element=w266:string[])  [unwired: 1 in]
        n99 = Index Array(array=w266, index=0 ("索引")) -> (element=w264:string)
        n100 = Format Into String(format string="delete from t_sample_set \nwhere time_sample_set_id='%s';", w264) -> (resulting string=w263:string)  [unwired: 2 in, 1 out]
        n101 = call "deleteData.vi"("SQL query"=w263) -> ()  [unwired: 10 in, 1 out]
        n102 = call <vilib>:"Add State(s) to Queue__JKI_lib_State_Machine.vi"("State(s) in (\"\")"=w273) -> ("States Out"=w272:string)  [unwired: 14 in]
      }
      frame "TimeSample:ModifyTimeSampleDlg" {
        # "Your code here.\n(You can make a copy of, or modify, this frame)"
        n103 = Unbundle By Name(w294) -> ("Row"=w298:i32)
        n104 = property on="定时采样设置" class="MCListbox (严格)"() -> ("ItemNames"=w299:string[][])  [unwired: 2 in, 2 out]
        n105 = Index Array(array=w299, index (row)=w298) -> (element=w292:string[])  [unwired: 1 in]
        n106 = Index Array(array=w292, index=8 ("索引")) -> (element=w278:string)
        n107 = Index Array(array=w292, index=5 ("索引")) -> (element=w281:string)
        n108 = Index Array(array=w292, index=7 ("索引")) -> (element=w279:string)
        n109 = Index Array(array=w292, index=3 ("索引")) -> (element=w277:string)
        n110 = Index Array(array=w292, index=4 ("索引")) -> (element=w275:string)
        n111 = Index Array(array=w292, index=1 ("索引")) -> (element=w283:string)
        n112 = Index Array(array=w292, index=6 ("索引")) -> (element=w280:string)
        n113 = Index Array(array=w292, index=2 ("索引")) -> (element=w282:string)
        n114 = Decimal String To Number(string=w275) -> (number=w274:i32)  [unwired: 2 in, 1 out]
        n115 = Decimal String To Number(string=w277) -> (number=w276:i32)  [unwired: 2 in, 1 out]
        n116 = Index Array(array=w292, index=0 ("索引")) -> (element=w296:string)
        "编号" <- w296
        n117 = Unbundle By Name(w294) -> ("定时采样信息"=w293:T1)
        n118 = Bundle By Name(cluster=w293, "检测区域"=w283, "时"=w276, "分钟"=w274, "供电位置"=w282, "是否启动"=w281, "备注"=w278, "电源电压"=w280, "电源频率"=w279) -> (w295:T1)
        n119 = call "TimeSampleDlgModify.vi"("序号"=w296, "定时采样信息in"=w295) -> ()  [unwired: 9 in, 1 out]
        n120 = call <vilib>:"Add State(s) to Queue__JKI_lib_State_Machine.vi"("State(s) in (\"\")"=w302) -> ("States Out"=w301:string)  [unwired: 14 in]
      }
      frame "TimeSample:NewTimeSampleDlg" {
        # "Your code here.\n(You can make a copy of, or modify, this frame)"
        n121 = call "TimeSampleDlgg.vi"() -> ("定时采样信息"=w303:T1)  [unwired: 11 in]
        n122 = Bundle By Name(cluster=w305, "定时采样信息"=w303) -> (w304:T4)
        n123 = call <vilib>:"Add State(s) to Queue__JKI_lib_State_Machine.vi"("State(s) in (\"\")"=w308) -> ("States Out"=w307:string)  [unwired: 14 in]
      }
    }
  }
  "定时采样out" <- "定时采样设置"
